vi "Configuration Window.vi"(8 "error in (no error)":errorcluster, 11 "FP-TC-Shared":refnum<class "FP-TC-Shared.lvclass">) -> (0 "error out":errorcluster, 3 "FP-TC-Shared out":refnum<class "FP-TC-Shared.lvclass">)   [LabVIEW 2019, in "FP-TC-Shared.lvclass"]
uses:
  FP-TC-Shared.lvclass
  typedefs/LC Type--Enum.ctl
  FP-TC-Shared.lvclass/FP-TC-Shared.ctl
panel:
  in  "Paths":string
  in  "LC Type":T1
  in  "Cancel":bool
  in  "OK":bool
  # "Confirm or Make Changes:"
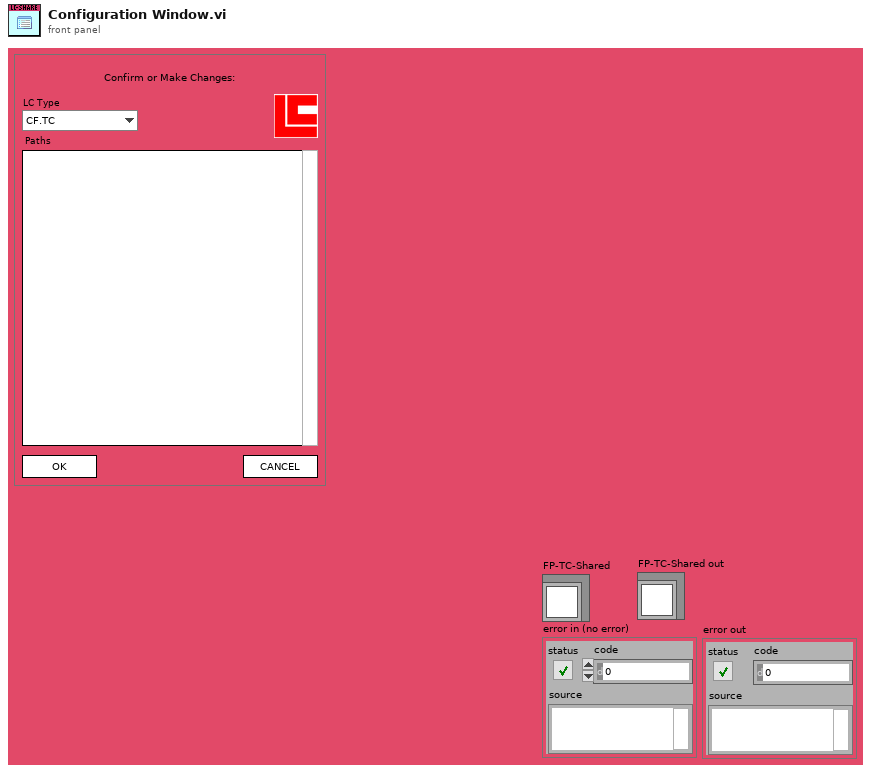
[diagram p1: front panel]
types:
  T1 = typedef "FP-TC-Shared.lvclass/LC Type--Enum.ctl" = enum16{"CF.TC", "CF.TC.Z", "CF.FP", "MNK.TC", "MNK.TC.Z", "MNK.FP"}
  T2 = enum32{"Invalid", "Standard", "Closed", "Hidden", "Minimized", "Maximized"}
  T3 = enum32{"invalid app kind", "Development System", "Run Time System", "Student Edition", "Embedded LabVIEW", "Evaluation", "Custom"}
  T4 = cluster{"Core":cluster{"Current VI Reference":refnum<vi>, "Close Panel on Exit?":bool}, "FP-TC-Shared out":refnum<class "FP-TC-Shared.lvclass">}
  T5 = cluster{"Current VI Reference":refnum<vi>, "Close Panel on Exit?":bool}
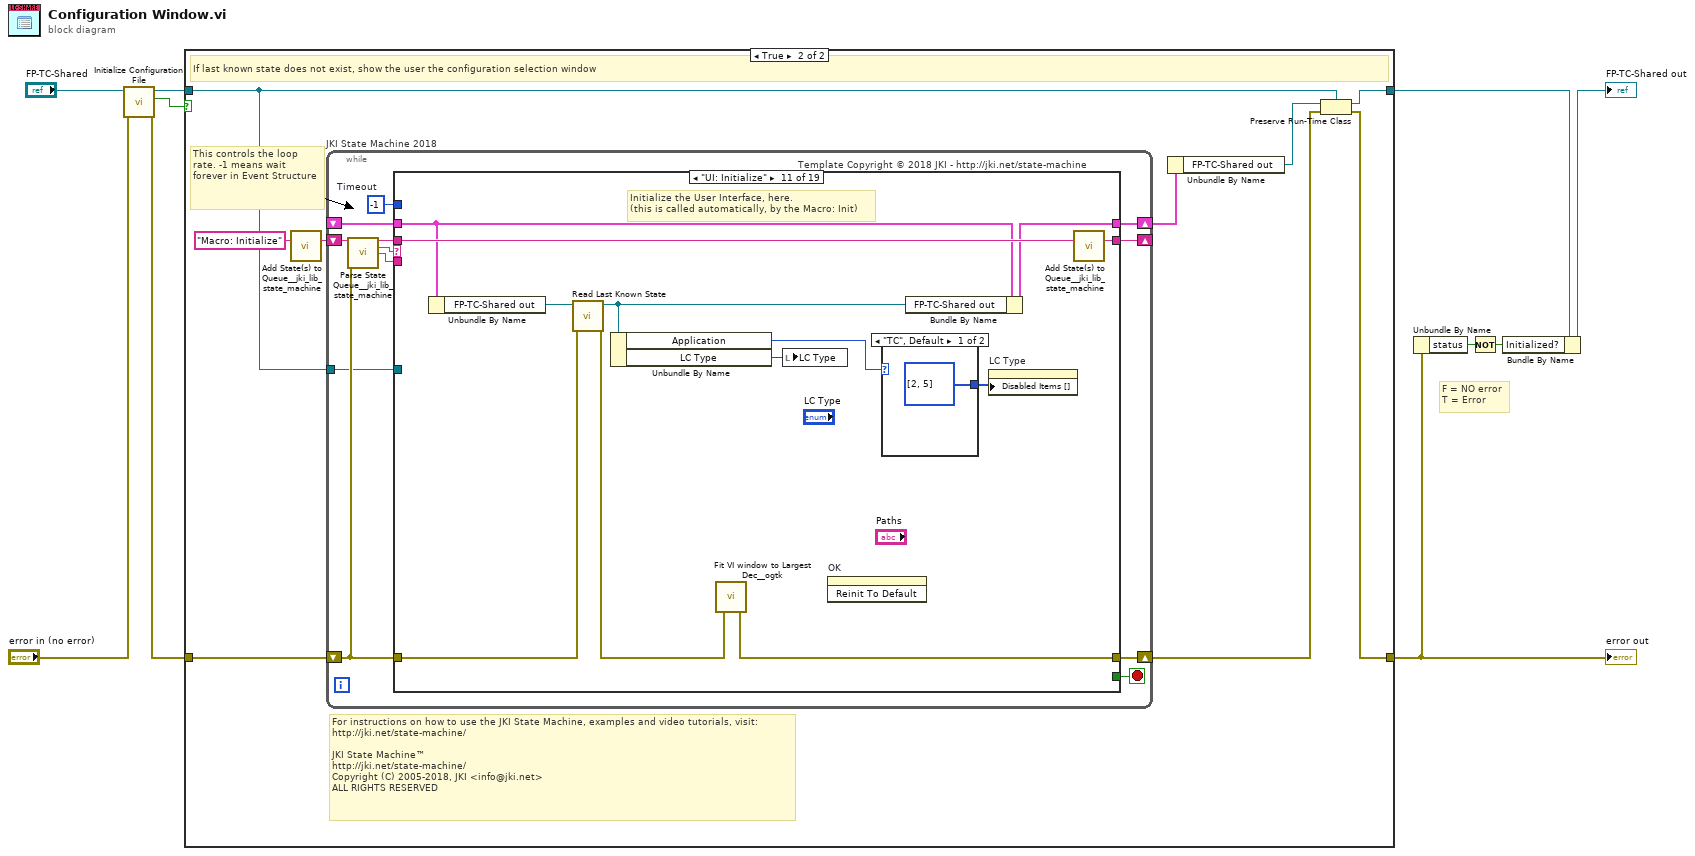
[diagram p0: block diagram]
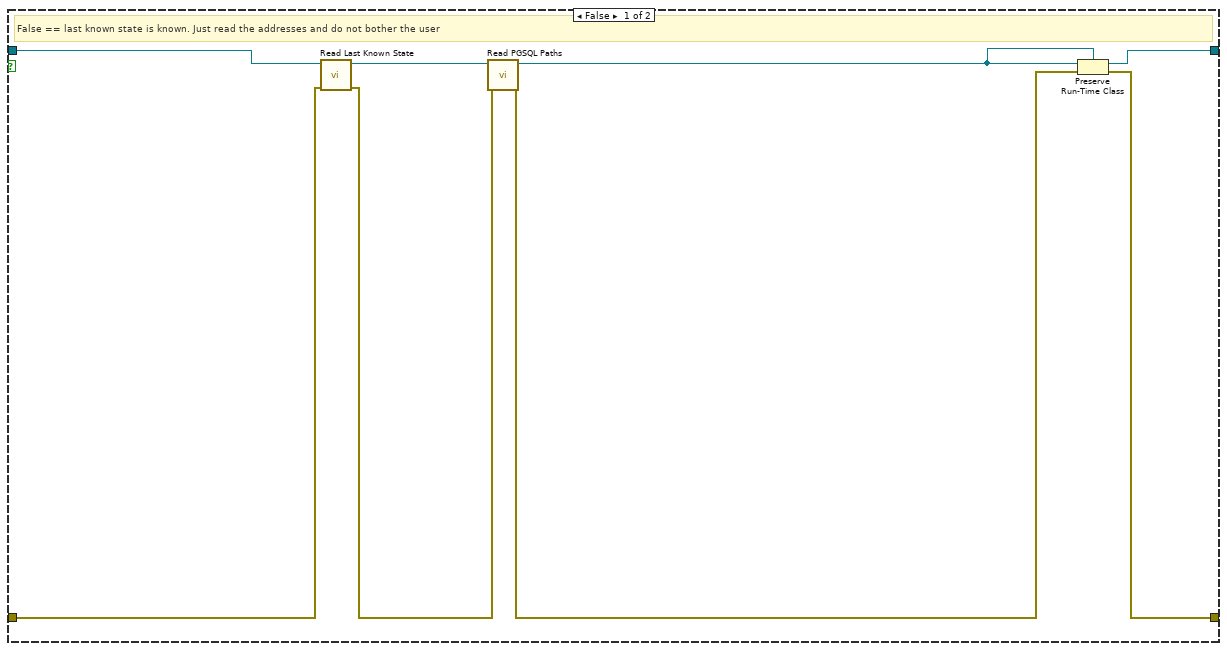
[diagram p2: hidden frame]
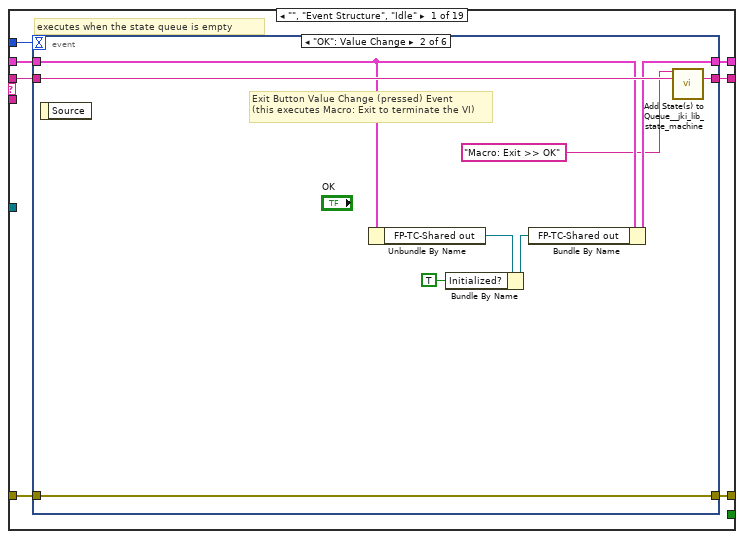
[diagram p3: hidden frame]
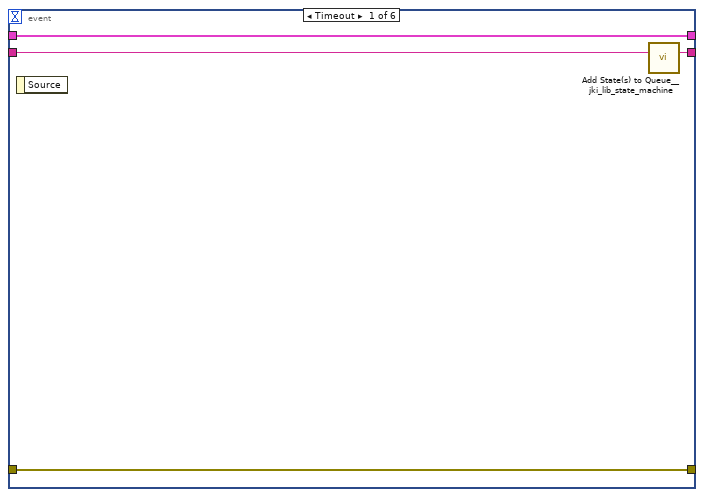
[diagram p4: hidden frame]
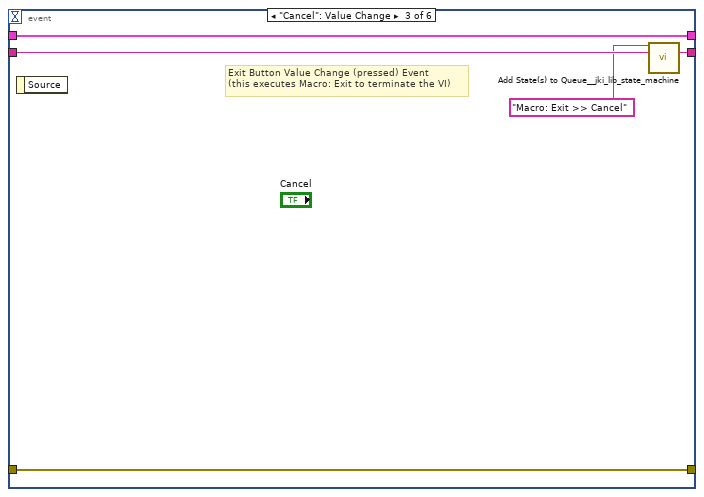
[diagram p5: hidden frame]
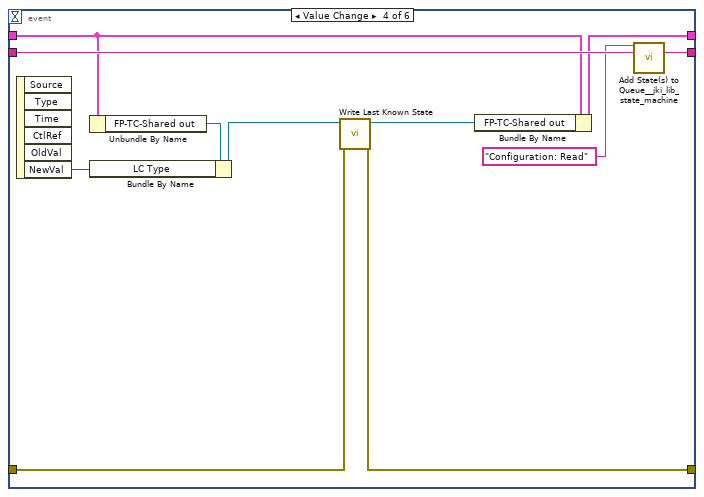
[diagram p6: hidden frame]
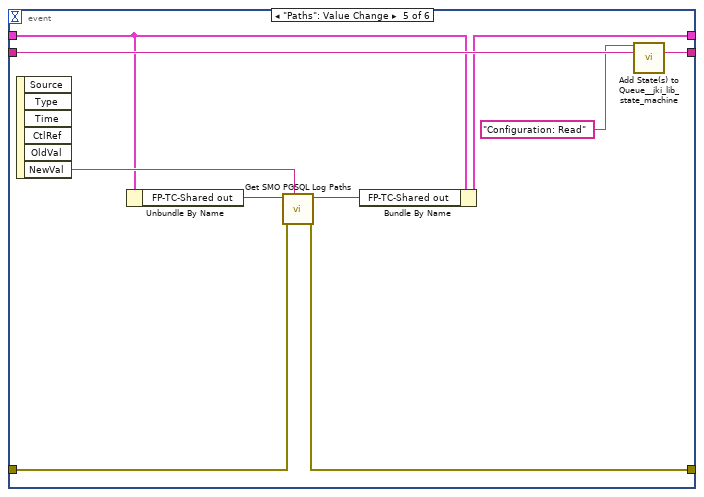
[diagram p7: hidden frame]
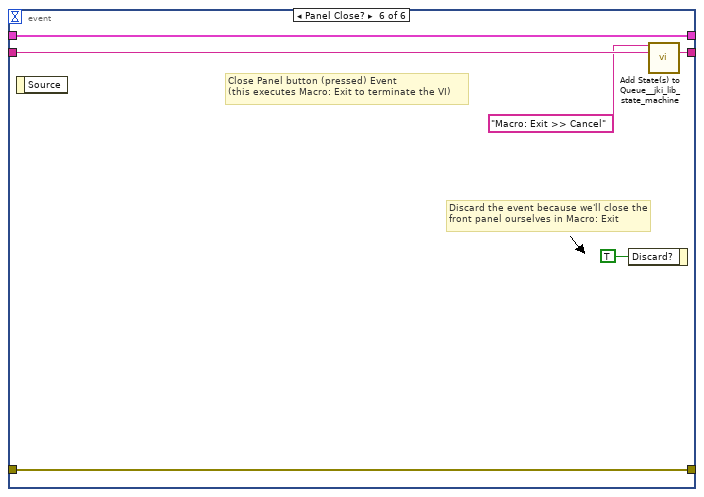
[diagram p8: hidden frame]
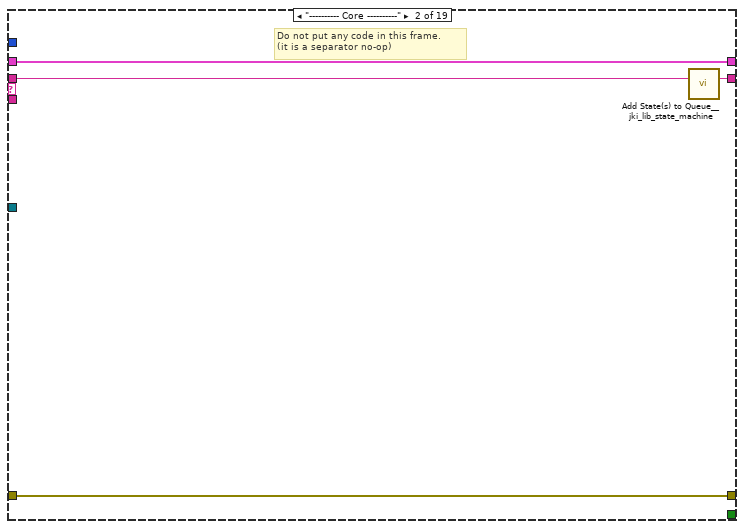
[diagram p9: hidden frame]
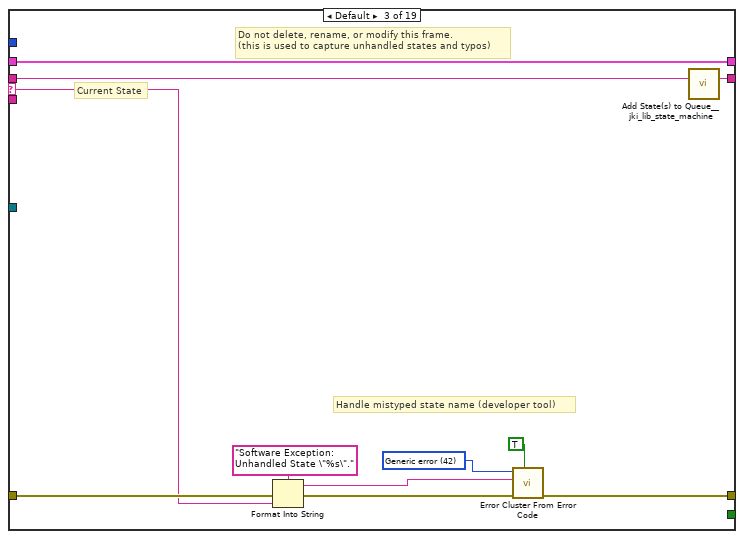
[diagram p10: hidden frame]
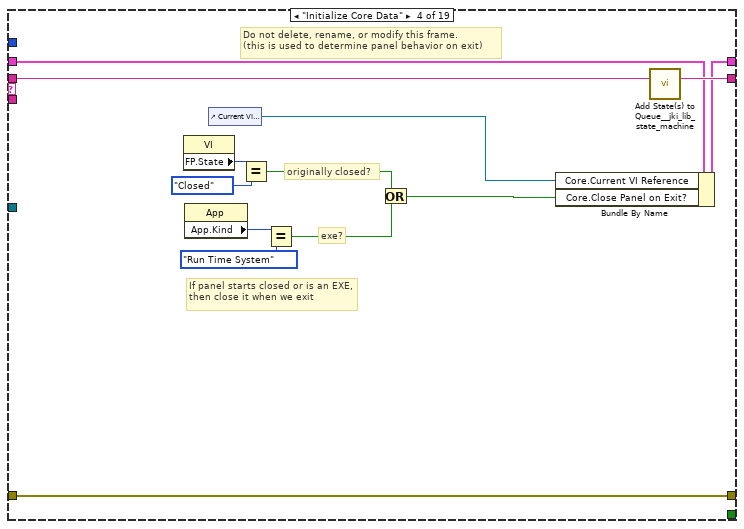
[diagram p11: hidden frame]
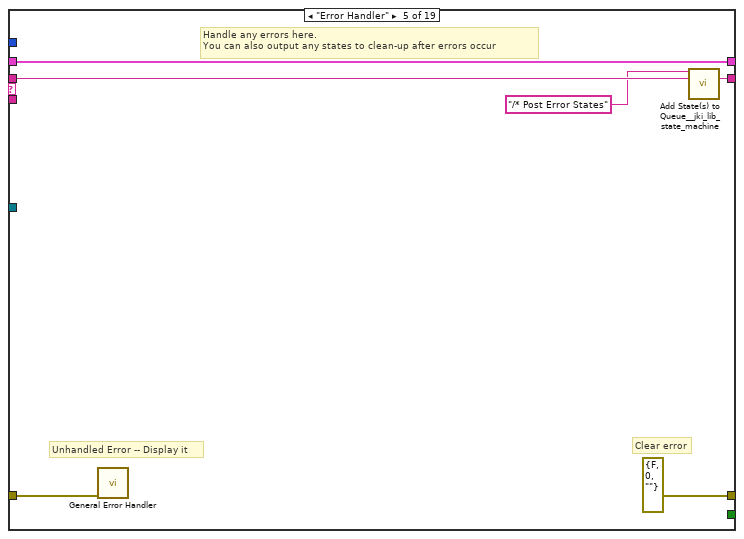
[diagram p12: hidden frame]
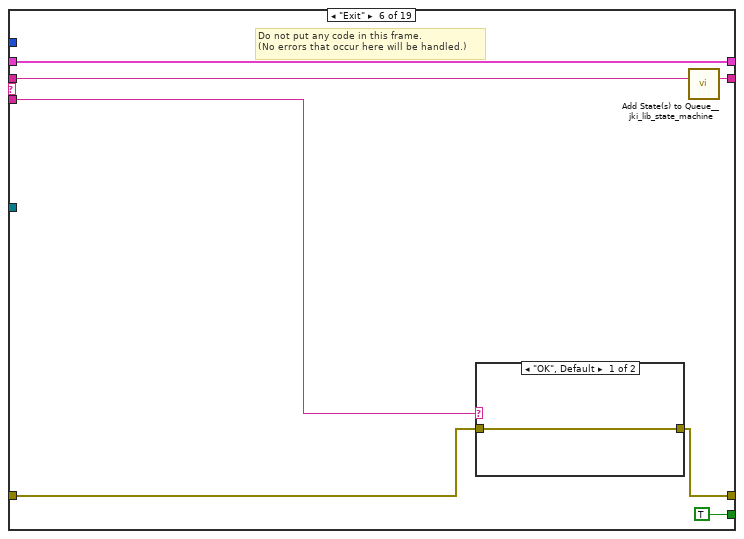
[diagram p13: hidden frame]
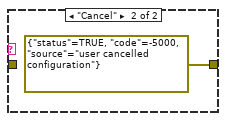
[diagram p14: hidden frame]
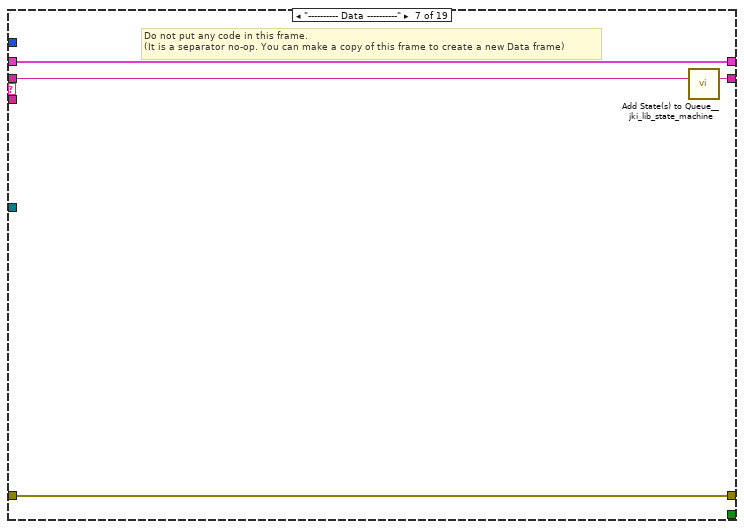
[diagram p15: hidden frame]
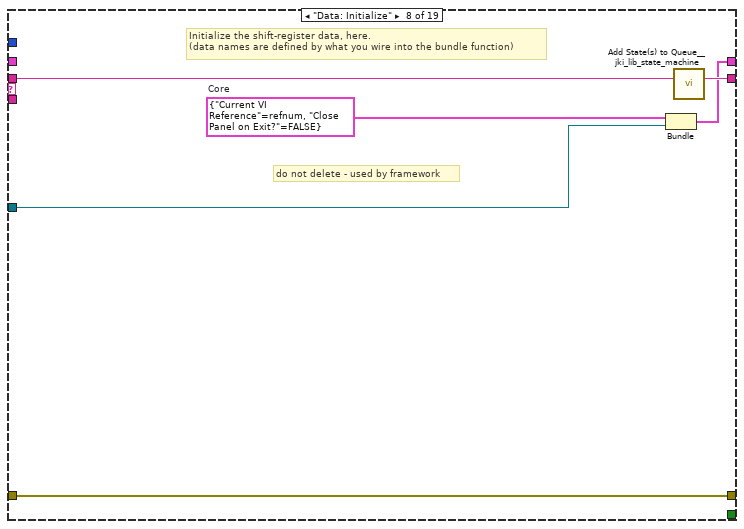
[diagram p16: hidden frame]
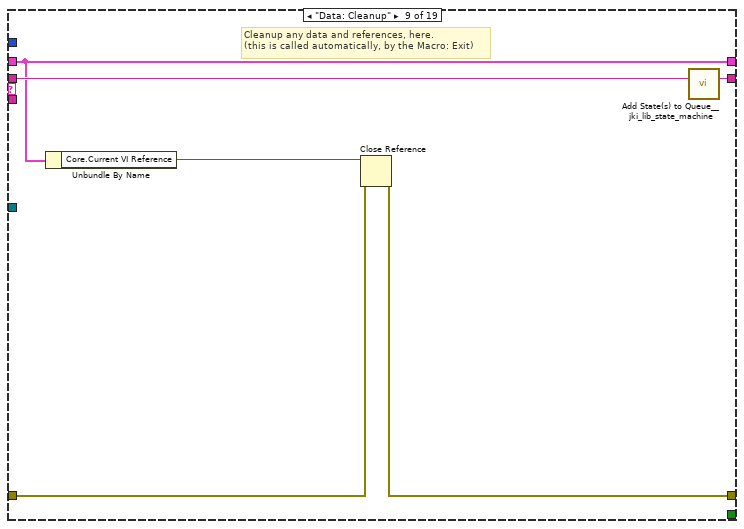
[diagram p17: hidden frame]
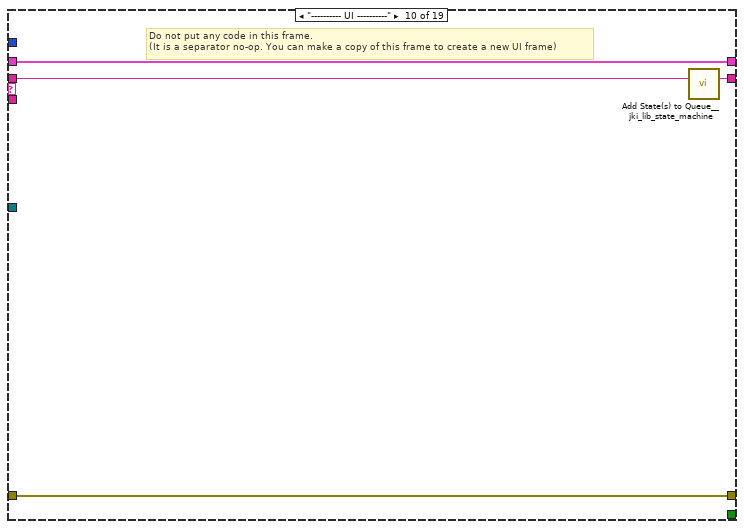
[diagram p18: hidden frame]
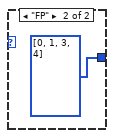
[diagram p19: hidden frame]
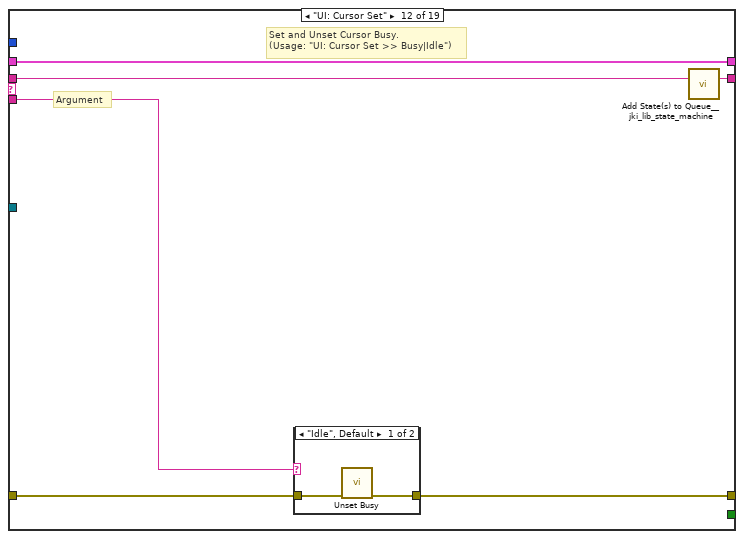
[diagram p20: hidden frame]
diagram:
  # "F = NO error\nT = Error"
  n1 = call "Initialize Configuration File.vi"("error in (no error)"="error in (no error)", "FP-TC-Shared in"="FP-TC-Shared") -> ("error out"=w9:errorcluster, "Last State Unknown"=w6:bool, "FP-TC-Shared out"=w7:refnum<class "FP-TC-Shared.lvclass">)  [unwired: 7 in]
  n2 = case shown="True" w6 {
    tunnel: w9 -> [w12 w25]
    tunnel: w7 -> [w14 w24]
    tunnel: [w16 w21] -> w3
    tunnel: [w18 w23] -> w2
    frame False {
      # "False == last known state is known. Just read the addresses and do not bother the user"
      n3 = call "Read Last Known State.vi"("error in (no error)"=w12, "FP-TC-Shared in"=w14) -> ("error out"=w11:errorcluster, "FP-TC-Shared out"=w13:refnum<class "FP-TC-Shared.lvclass">)  [unwired: 8 in]
      n4 = call "Read PGSQL Paths.vi"("error in (no error)"=w11, "FP-TC-Shared in"=w13) -> ("error out"=w17:errorcluster, "FP-TC-Shared out"=w15:refnum<class "FP-TC-Shared.lvclass">)  [unwired: 8 in]
      n5 = Preserve Run-Time Class(object in=w15, error in=w17, 2:w15) -> (object out=w18:refnum<class "FP-TC-Shared.lvclass">, error out=w16:errorcluster)
    }
    frame True {
      # "For instructions on how to use the JKI State Machine, examples and video tutorials, visit:\nhttp://jki.net/state-machine/\n\nJKI State Machine™\nhttp://jki.net/state-machine/\nCopyright (C) 2005-2018, JKI <info@jki.net>\nALL RIGHTS RESERVED"
      # "This controls the loop rate. -1 means wait forever in Event Structure"
      # "If last known state does not exist, show the user the configuration selection window"
      n6 = call <vilib>:"Add State(s) to Queue__jki_lib_state_machine.vi"("State(s) in (\"\")"="Macro: Initialize") -> ("States Out"=w27:string)  [unwired: 14 in]
      n7 = while "JKI State Machine 2018" {
        shift-right: [w32] -> w20
        shift-left: _ -> [w31]
        shift-right: [w35] -> w22
        shift-left: w25 -> [w29]
        shift-right: [w34] -> _
        shift-left: w27 -> [w36]
        tunnel: w24 -> [w28]
        stop <- w33 stop-if-true
        w30 = -1  # Timeout
        # "Template Copyright © 2018 JKI - http://jki.net/state-machine"
        n8 = call <vilib>:"Parse State Queue__jki_lib_state_machine.vi"("State Queue"=w36, "Error In (no error)"=w29) -> ("Remaining States"=w38:string, "Current State"=w39:string, "Arguments"=w37:string)  [unwired: 11 in]
        n9 = case shown="\"UI: Initialize\"" w39 {
          selector: w39 -> [_ _ w96 _ _ _ _ _ _ _ _ _ _ _ _ _ _ _ _]
          tunnel: w38 -> [w46 w95 w100 w119 w125 w132 w138 w144 w150 w154 w166 w174 w185 w254 w259 w274 w278 w288 w296]
          tunnel: w37 -> [_ _ _ _ _ w128 _ _ _ _ _ w169 w179 _ _ w263 _ _ _]
          tunnel: w31 -> [w44 w92 w98 w112 w122 w130 w135 _ w145 w151 w161 w172 w181 w251 w256 w271 w275 w284 w292]
          tunnel: [w43 w93 w102 w116 errorcluster {"status"=FALSE, "code"=0, "source"=""} ("error out") w126 w136 w140 w146 w152 w164 w170 w182 w252 w257 w272 w276 w281 w289] -> w35
          tunnel: w29 -> [w42 w93 w101 w116 w121 w127 w136 w140 w147 w152 w157 w171 w183 w252 w257 w272 w276 w282 w289]
          tunnel: [w45 w94 w99 w118 w124 w131 w137 w143 w149 w153 w165 w173 w184 w253 w258 w273 w277 w287 w295] -> w34
          tunnel: [_ _ _ _ _ TRUE _ _ _ _ _ _ _ _ _ _ _ _ _] -> w33
          tunnel: [w41 w92 w98 w117 w122 w130 w135 w142 w145 w151 w160 w172 w181 w251 w256 w271 w275 w285 w291] -> w32
          tunnel: w30 -> [w40 _ _ _ _ _ _ _ _ _ _ _ _ _ _ _ _ _ _]
          tunnel: w28 -> [_ _ _ _ _ _ _ w139 _ _ _ _ _ _ _ _ _ _ _]
          frame "", "Event Structure", "Idle" {
            # "executes when the state queue is empty"
            n10 = event shown="[1] \"OK\": Value Change" {
              selector: _ -> [_ _ _ _ _ _]
              dyn-events: _ -> [_ _ _ _ _ _]
              timeout: w40 -> [_ _ _ _ _ _]
              tunnel: w46 -> [w50 w59 w64 w74 w84 w91]
              tunnel: [w49 w58 w63 w75 w85 w90] -> w45
              tunnel: w44 -> [w47 w53 w60 w71 w76 w88]
              tunnel: [w48 w57 w62 w67 w80 w89] -> w43
              tunnel: w42 -> [w48 w57 w62 w68 w79 w89]
              tunnel: [w47 w54 w60 w72 w77 w88] -> w41
              event Timeout {
                n11 = event-data() -> ()  [unwired: 1 in, 1 out]
                n12 = call <vilib>:"Add State(s) to Queue__jki_lib_state_machine.vi"("State(s) in (\"\")"=w50) -> ("States Out"=w49:string)  [unwired: 14 in]
              }
              event "OK": Value Change {
                # "Exit Button Value Change (pressed) Event\n(this executes Macro: Exit to terminate the VI)"
                n13 = event-data() -> ()  [unwired: 1 in, 1 out]
                n14 = Unbundle By Name(w53) -> ("FP-TC-Shared out"=w56:refnum<class "FP-TC-Shared.lvclass">)
                n15 = Bundle By Name(cluster=w56, "Initialized?"=TRUE) -> (w55:refnum<class "FP-TC-Shared.lvclass">)
                n16 = Bundle By Name(cluster=w53, "FP-TC-Shared out"=w55) -> (w54:T4)
                n17 = call <vilib>:"Add State(s) to Queue__jki_lib_state_machine.vi"("State(s) in Front (\"\")"="Macro: Exit >> OK", "State(s) in (\"\")"=w59) -> ("States Out"=w58:string)  [unwired: 13 in]
              }
              event "Cancel": Value Change {
                # "Exit Button Value Change (pressed) Event\n(this executes Macro: Exit to terminate the VI)"
                n18 = event-data() -> ()  [unwired: 1 in, 1 out]
                n19 = call <vilib>:"Add State(s) to Queue__jki_lib_state_machine.vi"("State(s) in Front (\"\")"="Macro: Exit >> Cancel", "State(s) in (\"\")"=w64) -> ("States Out"=w63:string)  [unwired: 13 in]
              }
              event Value Change {
                n20 = event-data() -> ("NewVal"=w70:T1)  [unwired: 1 in, 5 out]
                n21 = Unbundle By Name(w71) -> ("FP-TC-Shared out"=w69:refnum<class "FP-TC-Shared.lvclass">)
                n22 = Bundle By Name(cluster=w69, "LC Type"=w70) -> (w65:refnum<class "FP-TC-Shared.lvclass">)
                n23 = call "Write Last Known State.vi"("error in (no error)"=w68, "FP-TC-Shared in"=w65) -> ("error out"=w67:errorcluster, "FP-TC-Shared out"=w66:refnum<class "FP-TC-Shared.lvclass">)  [unwired: 8 in]
                n24 = Bundle By Name(cluster=w71, "FP-TC-Shared out"=w66) -> (w72:T4)
                n25 = call <vilib>:"Add State(s) to Queue__jki_lib_state_machine.vi"("State(s) in Front (\"\")"="Configuration: Read" ("State(s) in Front (\"\")"), "State(s) in (\"\")"=w74) -> ("States Out"=w75:string)  [unwired: 13 in]
              }
              event "Paths": Value Change {
                n26 = event-data() -> ("NewVal"=w81:string)  [unwired: 1 in, 5 out]
                n27 = Unbundle By Name(w76) -> ("FP-TC-Shared out"=w82:refnum<class "FP-TC-Shared.lvclass">)
                n28 = call-dynamic "Get SMO PGSQL Log Paths.vi"("Default Paths"=w81, "error in (no error)"=w79, "FP-TC-Shared in"=w82) -> ("error out"=w80:errorcluster, "FP-TC-Shared out"=w78:refnum<class "FP-TC-Shared.lvclass">)  [unwired: 6 in, 1 out]
                n29 = Bundle By Name(cluster=w76, "FP-TC-Shared out"=w78) -> (w77:T4)
                n30 = call <vilib>:"Add State(s) to Queue__jki_lib_state_machine.vi"("State(s) in Front (\"\")"="Configuration: Read" ("State(s) in Front (\"\")"), "State(s) in (\"\")"=w84) -> ("States Out"=w85:string)  [unwired: 13 in]
              }
              event Panel Close? {
                # "Discard the event because we'll close the front panel ourselves in Macro: Exit"
                # "Close Panel button (pressed) Event\n(this executes Macro: Exit to terminate the VI)"
                n31 = event-data() -> ()  [unwired: 1 in, 1 out]
                n32 = event-data("Discard?"=TRUE) -> ()  [unwired: 1 in, 1 out]
                n33 = call <vilib>:"Add State(s) to Queue__jki_lib_state_machine.vi"("State(s) in Front (\"\")"="Macro: Exit >> Cancel", "State(s) in (\"\")"=w91) -> ("States Out"=w90:string)  [unwired: 13 in]
              }
            }
          }
          frame "---------- Core ----------" {
            # "Do not put any code in this frame.\n(it is a separator no-op)"
            n34 = call <vilib>:"Add State(s) to Queue__jki_lib_state_machine.vi"("State(s) in (\"\")"=w95) -> ("States Out"=w94:string)  [unwired: 14 in]
          }
          frame Default {
            w105 = 42 items=["No error", "Argument error", "Memory is full", "Out of zone", "End of file", "File already open", "Generic file I/O error", "File not found", "File permission error", "Disk is full", "Duplicate path", "Too many files open", "System feature not enabled", "Resource file not found", "Cannot add resource", "Resource not found", "Image not found", "Image memory error", "Pen does not exist", "Config type invalid", "Config token not found", "Config parse error", "Config memory error", "Bad external code format", "Bad external code offset", "External code not present", "Null window", "Destroy window error", "Null menu", "Print aborted", "Bad print record", "Print driver error", "Windows error during printing", "Memory error during printing", "Print dialog error", "Generic print error", "Invalid device refnum", "Device not found", "Device parameter error", "Device unit error", "Cannot open device", "Device call aborted", "Generic error", "Cancelled by user", "Object ID too low", "Object ID too high", "Object not in heap", "Unknown heap", "Unknown object (invalid DefProc)", "Unknown object (DefProc not in table)", "Message out of range", "Invalid (null) method", "Unknown message", "Manager call not supported", "Bad address", "Network operation in progress", "Network operation timed out", "Connection is busy", "Network attribute not supported", "Network error", "Address in use", "System out of memory", "Connection aborted", "Connection refused", "Not connected", "Already connected", "Connection closed", "Initialization error (interapplication manager)", "Bad occurrence", "Wait on unbound occurrence handler", "Occurrence queue overflow", "Datalog type conflict", "Unused", "Unrecognized type (interapplication manager)", "Memory corrupt", "Failed to make temporary DLL", "Old CIN version", "Drag socket not found", "Failed to load drop-object", "Failed to register OLE object", "Failed to release OLE object", "Format specifier type mismatch", "Unknown format specifier", "Too few format specifiers", "Too many format specifiers", "Scan failed", "Newer CIN version", "Error converting to variant", "Runtime menu error", "Password tampered", "Variant attribute not found", "Incompatible variant data type", "Event data is not available", "Event Store is not present", "Occurrence is not found", "Event Queue is not created", "Event info is not available", "Refnum passed is NULL", "Error retrieving Class GUID", "Error retrieving CoClass GUID", "Error retrieving TypeLib GUID.", "Bad built application magic bytes.", "Specific driver is different from the specific driver associated with the Logical Name.", "There is no session opened to the class driver.", "Max Error", "MAX - Error with config objects", "MAX - Error loading configuration", "MAX - Group not supported"]
            # "Current State"
            # "Do not delete, rename, or modify this frame.\n(this is used to capture unhandled states and typos)"
            # "Handle mistyped state name (developer tool)"
            n35 = Format Into String(format string="Software Exception: Unhandled State \"%s\"." ("message"), error in=w101, w96) -> (resulting string=w104:string, error out=w103:errorcluster)  [unwired: 1 in]
            n36 = call <vilib>:"Error Cluster From Error Code.vi"("show call chain? (False)"=TRUE, "error in (no error)"=w103, "error message (\"\")"=w104, "error code (0)"=w105) -> ("error out"=w102:errorcluster)  [unwired: 5 in]
            n37 = call <vilib>:"Add State(s) to Queue__jki_lib_state_machine.vi"("State(s) in (\"\")"=w100) -> ("States Out"=w99:string)  [unwired: 14 in]
          }
          frame "Initialize Core Data" {
            # "Do not delete, rename, or modify this frame.\n(this is used to determine panel behavior on exit)"
            # "originally closed?"
            # "exe?"
            # "If panel starts closed or is an EXE, then close it when we exit"
            n38 = property class="VI"() -> ("FP.State"=w109:T2)  [unwired: 2 in, 2 out]
            n39 = property class="App"() -> ("App.Kind"=w115:T3)  [unwired: 2 in, 2 out]
            n40 = control-ref of="Current VI Reference"() -> (w110:refnum<vi>)
            n41 = Equal?(x=w109, y=T2."Closed" ("Front Panel Window:State")) -> (x = y?=w107:bool)
            n42 = Equal?(x=w115, y=T3."Run Time System" ("Application:Kind")) -> (x = y?=w113:bool)
            n43 = Or(x=w107, y=w113) -> (x .or. y?=w111:bool)
            n44 = Bundle By Name(cluster=w112, "Core.Current VI Reference"=w110, "Core.Close Panel on Exit?"=w111) -> (w117:T4)
            n45 = call <vilib>:"Add State(s) to Queue__jki_lib_state_machine.vi"("State(s) in (\"\")"=w119) -> ("States Out"=w118:string)  [unwired: 14 in]
          }
          frame "Error Handler" {
            # "Unhandled Error -- Display it"
            # "Handle any errors here.\nYou can also output any states to clean-up after errors occur"
            # "Clear error"
            n46 = call <vilib>:"General Error Handler.vi"("error in (no error)"=w121) -> ()  [unwired: 10 in, 5 out]
            n47 = call <vilib>:"Add State(s) to Queue__jki_lib_state_machine.vi"("State(s) in Front (\"\")"="/* Post Error States", "State(s) in (\"\")"=w125) -> ("States Out"=w124:string)  [unwired: 13 in]
          }
          frame "Exit" {
            # "Do not put any code in this frame.\n(No errors that occur here will be handled.)"
            n48 = case shown="\"OK\", Default" w128 {
              tunnel: w127 -> [w133 _]
              tunnel: [w133 errorcluster {"status"=TRUE, "code"=-5000, "source"="user cancelled configuration"} ("error in (no error)")] -> w126
              frame "OK", Default {
              }
              frame "Cancel" {
              }
            }
            n49 = call <vilib>:"Add State(s) to Queue__jki_lib_state_machine.vi"("State(s) in (\"\")"=w132) -> ("States Out"=w131:string)  [unwired: 14 in]
          }
          frame "---------- Data ----------" {
            # "Do not put any code in this frame.\n(It is a separator no-op. You can make a copy of this frame to create a new Data frame)"
            n50 = call <vilib>:"Add State(s) to Queue__jki_lib_state_machine.vi"("State(s) in (\"\")"=w138) -> ("States Out"=w137:string)  [unwired: 14 in]
          }
          frame "Data: Initialize" {
            w141 = T5 {"Current VI Reference"=refnum, "Close Panel on Exit?"=FALSE}  # Core
            # "do not delete - used by framework"
            # "Initialize the shift-register data, here.\n(data names are defined by what you wire into the bundle function)"
            n51 = Bundle("Core"=w141, "FP-TC-Shared out"=w139) -> (w142:T4)  [unwired: 1 in]
            n52 = call <vilib>:"Add State(s) to Queue__jki_lib_state_machine.vi"("State(s) in (\"\")"=w144) -> ("States Out"=w143:string)  [unwired: 14 in]
          }
          frame "Data: Cleanup" {
            # "Cleanup any data and references, here.\n(this is called automatically, by the Macro: Exit)"
            n53 = Unbundle By Name(w145) -> ("Core.Current VI Reference"=w148:refnum<vi>)
            n54 = Close Reference(reference=w148, error in (no error)=w147) -> (error out=w146:errorcluster)
            n55 = call <vilib>:"Add State(s) to Queue__jki_lib_state_machine.vi"("State(s) in (\"\")"=w150) -> ("States Out"=w149:string)  [unwired: 14 in]
          }
          frame "---------- UI ----------" {
            # "Do not put any code in this frame.\n(It is a separator no-op. You can make a copy of this frame to create a new UI frame)"
            n56 = call <vilib>:"Add State(s) to Queue__jki_lib_state_machine.vi"("State(s) in (\"\")"=w154) -> ("States Out"=w153:string)  [unwired: 14 in]
          }
          frame "UI: Initialize" {
            # "Initialize the User Interface, here.\n(this is called automatically, by the Macro: Init)"
            n57 = Unbundle By Name(w161) -> ("FP-TC-Shared out"=w163:refnum<class "FP-TC-Shared.lvclass">)
            n58 = call "Read Last Known State.vi"("error in (no error)"=w157, "FP-TC-Shared in"=w163) -> ("error out"=w158:errorcluster, "FP-TC-Shared out"=w159:refnum<class "FP-TC-Shared.lvclass">)  [unwired: 8 in]
            n59 = Unbundle By Name(w159) -> ("Application"=w156:enum16{"TC", "FP"}, "LC Type"=w162:T1)
            n60 = call <userlib>:"Fit VI window to Largest Dec__ogtk.vi"("error in (no error)"=w158) -> ("error out"=w164:errorcluster)  [unwired: 5 in, 1 out]
            n61 = local write "LC Type"(w162) -> ()
            n62 = invoke on="OK" class="Bool" method="Reinit To Default"() -> ()  [unwired: 3 in, 3 out]
            n63 = case shown="\"TC\", Default" w156 {
              tunnel: [i32[] [2, 5] ("Disabled Items []") i32[] [0, 1, 3, 4] ("Disabled Items []")] -> w155
              frame "TC", Default {
              }
              frame "FP" {
              }
            }
            n64 = Bundle By Name(cluster=w161, "FP-TC-Shared out"=w159) -> (w160:T4)
            n65 = property on="LC Type" class="Enum (strict)"("Disabled Items []"=w155) -> ()  [unwired: 2 in, 2 out]
            n66 = call <vilib>:"Add State(s) to Queue__jki_lib_state_machine.vi"("State(s) in (\"\")"=w166) -> ("States Out"=w165:string)  [unwired: 14 in]
          }
          frame "UI: Cursor Set" {
            # "Argument"
            # "Set and Unset Cursor Busy.\n(Usage: \"UI: Cursor Set >> Busy|Idle\")"
            n67 = case shown="\"Idle\", Default" w169 {
              tunnel: w171 -> [w176 w178]
              tunnel: [w175 w177] -> w170
              frame "Idle", Default {
                n68 = call <vilib>:"Unset Busy.vi"("error in (no error)"=w176) -> ("error out"=w175:errorcluster)  [unwired: 10 in]
              }
              frame "Busy" {
                n69 = call <vilib>:"Set Busy.vi"("error in (no error)"=w178) -> ("error out"=w177:errorcluster)  [unwired: 9 in, 1 out]
              }
            }
            n70 = call <vilib>:"Add State(s) to Queue__jki_lib_state_machine.vi"("State(s) in (\"\")"=w174) -> ("States Out"=w173:string)  [unwired: 14 in]
          }
          frame "UI: Front Panel State" {
            # "Argument"
            # "Set Front Panel Open or Closed\n(Usage: \"UI: Front Panel State >> Open|Close\")"
            n71 = Unbundle By Name(w181) -> ("Core.Current VI Reference"=w180:refnum<vi>)
            n72 = case shown="\"Maximize\", \"Maximized\"" w179 {
              tunnel: w183 -> [w191 w206 w217 w230 w243]
              tunnel: [w193 w207 w219 w232 w245] -> w182
              tunnel: w180 -> [w192 w204 w218 w231 w244]
              frame "Open", "Standard", Default {
                w186 = T2."Standard" ("State")
                n73 = property class="VI"(reference=w192, error in=w191) -> (reference out=w189:refnum<vi>, error out=w190:errorcluster, "FP.State"=w188:T2)
                n74 = Not Equal?(x=w188, y=w186) -> (x != y?=w187:bool)
                n75 = case shown="True" w187 {
                  tunnel: [w197 w199] -> w193
                  tunnel: w190 -> [w196 w199]
                  tunnel: w189 -> [w195 _]
                  tunnel: w186 -> [w194 _]
                  frame True {
                    n76 = invoke class="VI" method="FP.Open"(reference=w195, error in=w196, "Activate"=TRUE, "State"=w194) -> (error out=w197:errorcluster)  [unwired: 1 in, 4 out]
                  }
                  frame False {
                  }
                }
              }
              frame "Close", "Closed" {
                n77 = property class="VI"(reference=w204, error in=w206) -> (reference out=w203:refnum<vi>, error out=w205:errorcluster, "FP.State"=w201:T2)
                n78 = Not Equal?(x=w201, y=T2."Closed" ("Front Panel Window:State")) -> (x != y?=w200:bool)
                n79 = case shown="True" w200 {
                  tunnel: [w208 w211] -> w207
                  tunnel: w205 -> [w208 w210]
                  tunnel: w203 -> [_ w209]
                  frame False {
                  }
                  frame True {
                    n80 = invoke class="VI" method="FP.Close"(reference=w209, error in=w210) -> (error out=w211:errorcluster)  [unwired: 1 in, 2 out]
                  }
                }
              }
              frame "Hidden", "Hide" {
                w212 = T2."Hidden" ("State")
                n81 = property class="VI"(reference=w218, error in=w217) -> (reference out=w215:refnum<vi>, error out=w216:errorcluster, "FP.State"=w214:T2)
                n82 = Not Equal?(x=w214, y=w212) -> (x != y?=w213:bool)
                n83 = case shown="True" w213 {
                  tunnel: [w223 w224] -> w219
                  tunnel: w216 -> [w222 w224]
                  tunnel: w215 -> [w221 _]
                  tunnel: w212 -> [w220 _]
                  frame True {
                    n84 = invoke class="VI" method="FP.Open"(reference=w221, error in=w222, "State"=w220) -> (error out=w223:errorcluster)  [unwired: 2 in, 4 out]
                  }
                  frame False {
                  }
                }
              }
              frame "Minimize", "Minimized" {
                w225 = T2."Minimized" ("State")
                n85 = property class="VI"(reference=w231, error in=w230) -> (reference out=w228:refnum<vi>, error out=w229:errorcluster, "FP.State"=w227:T2)
                n86 = Not Equal?(x=w227, y=w225) -> (x != y?=w226:bool)
                n87 = case shown="True" w226 {
                  tunnel: [w236 w237] -> w232
                  tunnel: w229 -> [w235 w237]
                  tunnel: w228 -> [w234 _]
                  tunnel: w225 -> [w233 _]
                  frame True {
                    n88 = invoke class="VI" method="FP.Open"(reference=w234, error in=w235, "State"=w233) -> (error out=w236:errorcluster)  [unwired: 2 in, 4 out]
                  }
                  frame False {
                  }
                }
              }
              frame "Maximize", "Maximized" {
                w238 = T2."Maximized" ("State")
                n89 = property class="VI"(reference=w244, error in=w243) -> (reference out=w241:refnum<vi>, error out=w242:errorcluster, "FP.State"=w240:T2)
                n90 = Not Equal?(x=w240, y=w238) -> (x != y?=w239:bool)
                n91 = case shown="True" w239 {
                  tunnel: [w249 w250] -> w245
                  tunnel: w242 -> [w248 w250]
                  tunnel: w241 -> [w247 _]
                  tunnel: w238 -> [w246 _]
                  frame True {
                    n92 = invoke class="VI" method="FP.Open"(reference=w247, error in=w248, "State"=w246) -> (error out=w249:errorcluster)  [unwired: 2 in, 4 out]
                  }
                  frame False {
                  }
                }
              }
            }
            n93 = call <vilib>:"Add State(s) to Queue__jki_lib_state_machine.vi"("State(s) in (\"\")"=w185) -> ("States Out"=w184:string)  [unwired: 14 in]
          }
          frame "---------- Macro ----------" {
            # "Do not put any code in this frame.\n(It is a separator no-op. You can make a copy of this frame to create a new Macro frame)"
            n94 = call <vilib>:"Add State(s) to Queue__jki_lib_state_machine.vi"("State(s) in (\"\")"=w254) -> ("States Out"=w253:string)  [unwired: 14 in]
          }
          frame "Macro: Initialize" {
            w255 = "Data: Initialize\nInitialize Core Data\nUI: Initialize\nUI: Front Panel State >> Open\nConfiguration: Read"  # Data: Initialize Initialize Core Data UI: Initialize UI: Front Panel State >> Open Configuration: Read
            # "Initialization Macro\n(This is called once, when the VI starts)"
            n95 = call <vilib>:"Add State(s) to Queue__jki_lib_state_machine.vi"("State(s) in Front (\"\")"=w255, "State(s) in (\"\")"=w259) -> ("States Out"=w258:string)  [unwired: 13 in]
          }
          frame "Macro: Exit" {
            # "Exit Macro\n(This is called once, when the VI exits)"
            n96 = Unbundle By Name(w271) -> ("Core.Close Panel on Exit?"=w270:bool)
            n97 = call <vilib>:"Build State String with Arguments__JKI_lib_State_Machine.vi"("Arguments (\"\")"=w263, "State"="Exit") -> ("State with Arguments"=w261:string)  [unwired: 4 in]
            n98 = Select(t="UI: Front Panel State >> Close", s=w270, f="") -> (s? t:f=w267:string)
            n99 = call <vilib>:"Add State(s) to Queue__jki_lib_state_machine.vi"("State(s) in Front (\"\")"="Data: Cleanup", "State(s) at Back (\"\")"=w261) -> ("States Out"=w260:string)  [unwired: 13 in]
            n100 = call <vilib>:"Add State(s) to Queue__jki_lib_state_machine.vi"("State(s) in Front (\"\")"="Configuration: Write", "State(s) in (\"\")"=w267, "State(s) at Back (\"\")"=w260) -> ("States Out"=w266:string)  [unwired: 12 in]
            n101 = call <vilib>:"Add State(s) to Queue__jki_lib_state_machine.vi"("State(s) in Front (\"\")"=w266, "State(s) in (\"\")"=w274) -> ("States Out"=w273:string)  [unwired: 13 in]
          }
          frame "---------- Configuration ----------" {
            # "Template Separator\n(You can make a copy of, or modify, this frame)"
            n102 = call <vilib>:"Add State(s) to Queue__jki_lib_state_machine.vi"("State(s) in (\"\")"=w278) -> ("States Out"=w277:string)  [unwired: 14 in]
          }
          frame "Configuration: Read" {
            # "Your code here.\n(You can make a copy of, or modify, this frame)"
            n103 = Unbundle By Name(w284) -> ("FP-TC-Shared out"=w283:refnum<class "FP-TC-Shared.lvclass">)
            n104 = Unbundle By Name(w283) -> ("LC Type"=w286:T1)
            n105 = call "Read PGSQL Paths.vi"("error in (no error)"=w282, "FP-TC-Shared in"=w283) -> ("error out"=w281:errorcluster, "FP-TC-Shared out"=w280:refnum<class "FP-TC-Shared.lvclass">)  [unwired: 8 in]
            n106 = Unbundle By Name(w280) -> ("Paths"=w279:string)
            n107 = local write "LC Type"(w286) -> ()
            n108 = local write "Paths"(w279) -> ()
            n109 = Bundle By Name(cluster=w284, "FP-TC-Shared out"=w280) -> (w285:T4)
            n110 = call <vilib>:"Add State(s) to Queue__jki_lib_state_machine.vi"("State(s) in (\"\")"=w288) -> ("States Out"=w287:string)  [unwired: 14 in]
          }
          frame "Configuration: Write" {
            n111 = local read "LC Type"() -> (w294:T1)
            n112 = Unbundle By Name(w292) -> ("FP-TC-Shared out"=w293:refnum<class "FP-TC-Shared.lvclass">)
            n113 = Bundle By Name(cluster=w293, "LC Type"=w294) -> (w290:refnum<class "FP-TC-Shared.lvclass">)
            n114 = Bundle By Name(cluster=w292, "FP-TC-Shared out"=w290) -> (w291:T4)
            n115 = call <vilib>:"Add State(s) to Queue__jki_lib_state_machine.vi"("State(s) in (\"\")"=w296) -> ("States Out"=w295:string)  [unwired: 14 in]
          }
        }
      }
      n116 = Unbundle By Name(w20) -> ("FP-TC-Shared out"=w19:refnum<class "FP-TC-Shared.lvclass">)
      n117 = Preserve Run-Time Class(object in=w19, error in=w22, 2:w24) -> (object out=w23:refnum<class "FP-TC-Shared.lvclass">, error out=w21:errorcluster)
    }
  }
  "error out" <- w3
  n118 = Unbundle By Name(w3) -> ("status"=w5:bool)
  n119 = Not(x=w5) -> (.not. x?=w4:bool)
  n120 = Bundle By Name(cluster=w2, "Initialized?"=w4) -> (→"FP-TC-Shared out":refnum<class "FP-TC-Shared.lvclass">)
